vi "OnGo.vi"(8 "error in":errorcluster, 9 "In Motion":refnum<vi>, 10 "UI":T1, 11 "CmdLib Out":refnum<k24>) -> (0 "error out":errorcluster)   [LabVIEW 2009]
uses:
  C:/Code/Apps/Utilities/Picomotor/PicomotorApp/Install/Samples/LabVIEW/Model 8742/LabVIEW 2009/CmdLib.dll
  Global Variables.vi
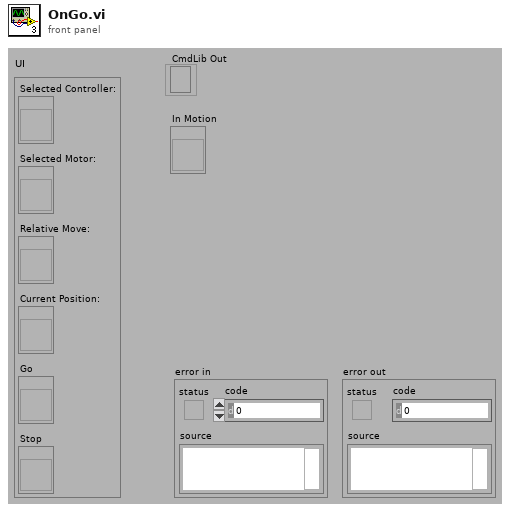
[diagram p1: front panel]
types:
  T1 = cluster{"Selected Controller:":refnum<vi>, "Selected Motor:":refnum<vi>, "Relative Move:":refnum<vi>, "Current Position:":refnum<vi>, "Go":refnum<vi>, "Stop":refnum<vi>}
  T2 = enum8{"Enabled", "Disabled", "Disabled and Grayed Out"}
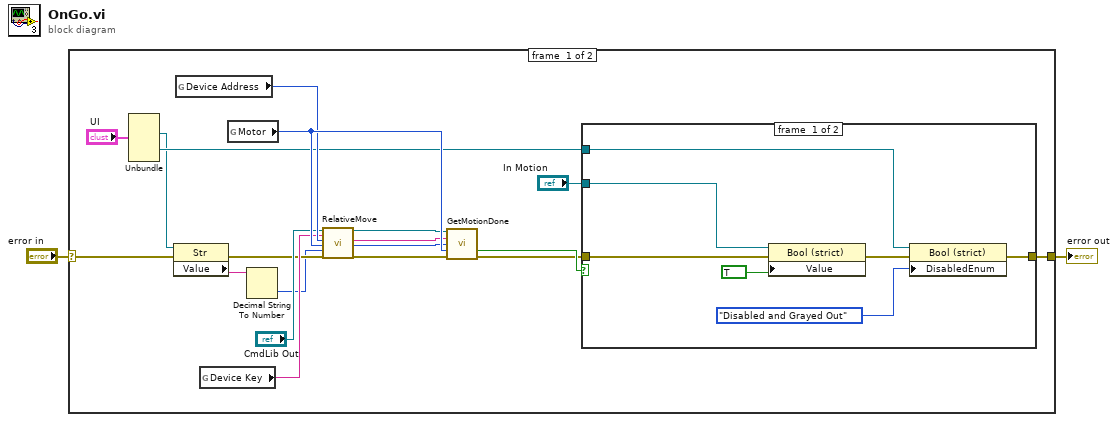
[diagram p0: block diagram]
diagram:
  n1 = case shown="No Error" "error in" {
    selector: "error in" -> [w6 w30]
    tunnel: [w13 w30] -> w2
    frame #0 {
      n2 = Unbundle("UI") -> ("Relative Move:"=w3:refnum<vi>, "Go"=w4:refnum<vi>)  [unwired: 4 out]
      n3 = property class="Str"(reference=w3, error in=w6) -> (error out=w9:errorcluster, "Value"=w7:string)  [unwired: 1 out]
      n4 = global read "Global Variables.vi" "Device Address"() -> (w12:i32)
      n5 = global read "Global Variables.vi" "Device Key"() -> (w11:string)
      n6 = global read "Global Variables.vi" "Motor"() -> (w19:i32)
      n7 = Decimal String To Number(string=w7) -> (number=w8:i32)  [unwired: 2 in, 1 out]
      n8 = call "RelativeMove.vi"("CmdLib In"="CmdLib Out", "DeviceKey In"=w11, "Device Address In"=w12, "Motor"=w19, "Relative Steps"=w8, "error in (no error)"=w9) -> ("CmdLib Out"=w16:refnum<k24>, "DeviceKey Out"=w17:string, "Device Address Out"=w18:i32, "error out"=w14:errorcluster)  [unwired: 10 in]
      n9 = call "GetMotionDone.vi"("CmdLib In"=w16, "DeviceKey In"=w17, "Device Address In"=w18, "Motor"=w19, "error in (no error)"=w14) -> ("Is Motion Done"=w20:bool, "error out"=w15:errorcluster)  [unwired: 6 in, 3 out]
      n10 = case shown="False" w20 {
        tunnel: [w22 w29] -> w13
        tunnel: w4 -> [w27 _]
        tunnel: w15 -> [w24 w29]
        tunnel: "In Motion" -> [w26 _]
        frame #0 {
          n11 = property class="Bool (strict)"(reference=w26, error in=w24, "Value"=TRUE) -> (error out=w23:errorcluster)  [unwired: 1 out]
          n12 = property class="Bool (strict)"(reference=w27, error in=w23, "DisabledEnum"=T2."Disabled and Grayed Out" ("Disabled")) -> (error out=w22:errorcluster)  [unwired: 1 out]
        }
        frame #1 {
        }
      }
    }
    frame #1 {
    }
  }
  "error out" <- w2
